vi "Add multiple points to Route.vi"(8 "Error In":errorcluster, 10 "Points":T1[](array[typedef]) {"Latitude" format="%#_10g"; "Longitude" format="%#_10g"}, 11 "Route Index":i32) -> (0 "Error Out":errorcluster)   [LabVIEW 2014]
uses:
  Lat Long Conversion/Controls/PointLatLon.ctl
  C:/Robotic Systems/Products/AgFalcon/Software/Ground Station/Data/Mapping DLL/GMap.NET.WindowsForms.dll
  Data/Mapping DLL/GMap.NET.WindowsForms.dll
  C:/Robotic Systems/Products/AgFalcon/Software/Ground Station/Data/Mapping DLL/GMap.NET.Core.dll
  Data/Mapping DLL/GMap.NET.Core.dll
  Reference/SubVI/GMap DLL Refernce.vi
  Reference/SubVI/Main Map Control Refernce.vi
  Missions/FGVs/Currently Selected Virtual WP/Methods/Set Current Virtual Waypoint.vi
  Application Support/Data Processing Queue/SubVI/Set Operations Queue.vi
  Missions/FGVs/Current Mission Distance/Methods/Set Mission Distance.vi
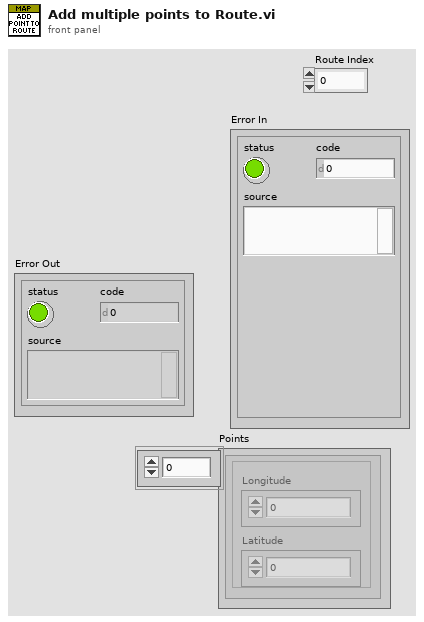
[diagram p1: front panel]
types:
  T1 = typedef "PointLatLon.ctl" = cluster{"Longitude":dbl, "Latitude":dbl}
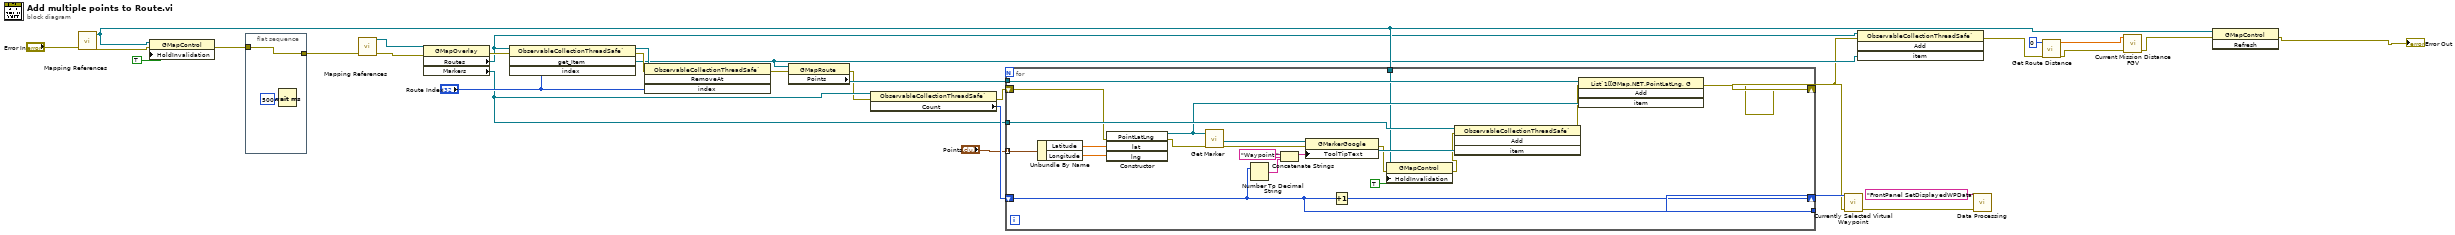
[diagram p0: block diagram]
diagram:
  n1 = call-poly "Mapping References.vi"("Error In"="Error In") -> ("Error Out"=w14:errorcluster, "GMap DLL Reference"=w10:refnum<k24>)  [unwired: 9 in]
  n2 = property class="GMapControl"(reference=w10, error in=w14, "HoldInvalidation"=TRUE) -> (error out=w11:errorcluster)  [unwired: 1 out]
  n3 = flat-sequence {
    tunnel: [w33] -> w12
    tunnel: w11 -> [w33]
    frame #0 {
      n4 = Wait (ms)(milliseconds to wait=u32 500) -> ()  [unwired: 1 out]
    }
  }
  n5 = call-poly "Mapping References.vi"("Error In"=w12) -> ("Error Out"=w25:errorcluster, "Main Map Reference"=w27:refnum<k24>)  [unwired: 9 in]
  n6 = property class="GMapOverlay"(reference=w27, error in=w25) -> (error out=w31:errorcluster, "Routes"=w9:refnum<k24>, "Markers"=w16:refnum<k24>)  [unwired: 1 out]
  n7 = invoke class="ObservableCollectionThreadSafe`" method="get_Item"(reference=w9, error in=w31, "index"="Route Index") -> (reference out=w29:refnum<k24>, error out=w30:errorcluster, "get_Item"=w7:refnum<k24>)  [unwired: 1 in, 1 out]
  n8 = invoke class="ObservableCollectionThreadSafe`" method="RemoveAt"(reference=w29, error in=w30, "index"="Route Index") -> (error out=w24:errorcluster)  [unwired: 1 in, 3 out]
  n9 = property class="GMapRoute"(reference=w7, error in=w24) -> (error out=w15:errorcluster, "Points"=w28:refnum<k24>)  [unwired: 1 out]
  n10 = property class="ObservableCollectionThreadSafe`"(reference=w16, error in=w15) -> (error out=w18:errorcluster, "Count"=w23:i32)  [unwired: 1 out]
  n11 = for {
    tunnel: w28 -> [w42]
    tunnel: w16 -> [w53]
    shift-right: [w34] -> w6
    shift-left: w18 -> [w40]
    shift-right: [w47] -> _
    shift-left: w23 -> [w46]
    tunnel: [w46] -> w20
    tunnel: "Points" -> [w45] mode=indexing
    tunnel: w10 -> [w37]
    n12 = Unbundle By Name(w45) -> ("Latitude"=w44:dbl, "Longitude"=w43:dbl)
    n13 = constructor class="PointLatLng"(error in=w40, "lat"=w44, "lng"=w43) -> (reference out=w41:refnum<k24>, error out=w48:errorcluster)  [unwired: 2 in, 3 out]
    n14 = call "Get Marker.vi"("Error In"=w48, "Point"=w41) -> ("error out"=w49:errorcluster, "new reference"=w55:refnum<k24>)  [unwired: 8 in]
    n15 = Number To Decimal String(number=w46) -> (decimal integer string=w52:string)  [unwired: 1 in]
    n16 = Concatenate Strings("Waypoint " ("string"), w52) -> (w50:string)
    n17 = property class="GMarkerGoogle"(reference=w55, error in=w49, "ToolTipText"=w50) -> (reference out=w54:refnum<k24>, error out=w36:errorcluster)
    n18 = Increment(x=w46) -> (x+1=w47:i32)
    n19 = property class="GMapControl"(reference=w37, error in=w36, "HoldInvalidation"=TRUE) -> (error out=w35:errorcluster)  [unwired: 1 out]
    n20 = invoke class="ObservableCollectionThreadSafe`" method="Add"(reference=w53, error in=w35, "item"=w54) -> (error out=w39:errorcluster)  [unwired: 1 in, 3 out]
    n21 = invoke class="List`1[[GMap.NET.PointLatLng, G" method="Add"(reference=w42, error in=w39, "item"=w41) -> (error out=w34:errorcluster)  [unwired: 1 in, 3 out]
  }
  n22 = call-poly "Currently Selected Virtual Waypoint.vi"("Error In"=w6, "Waypoint Index In"=w20) -> ("Error Out"=w21:errorcluster)  [unwired: 9 in]
  n23 = invoke class="ObservableCollectionThreadSafe`" method="Add"(reference=w9, error in=w6, "item"=w7) -> (error out=w5:errorcluster)  [unwired: 1 in, 3 out]
  n24 = call-poly "Data Processing.vi"("error in (no error)"=w21, "Command"="FrontPanel SetDisplayedWPData") -> ()  [unwired: 9 in, 1 out]
  n25 = call "Get Route Distance.vi"("Error In"=w5, "ROute Index"=0) -> ("error out"=w3:errorcluster, "Distance"=w2:dbl)  [unwired: 8 in]
  n26 = call-poly "Current Mission Distance FGV.vi"("Error In"=w3, "Distance In (km)"=w2) -> ("Error Out"=w1:errorcluster)  [unwired: 9 in]
  n27 = invoke class="GMapControl" method="Refresh"(reference=w10, error in=w1) -> (error out=→"Error Out":errorcluster)  [unwired: 1 in, 2 out]
